vi "Acquisition Message Loop.vi"(8 "error in (no error)":errorcluster, 9 "queue out":refnum<queue>, 10 "Data Notifier":refnum<notifier>, 11 "Message Queues":T1) -> (0 "error out":errorcluster)   [LabVIEW 2022 SP3, in "Acquisition.lvlib"]
doc: "Message loop for handling messages pertaining to the acquisition of data from the hardware."
uses:
  Acquisition.lvlib
  support/Message Queue/Message Cluster.ctl
  Acquisition State.ctl
  GlobalVariable/GlobalDisconnected.vi
  GlobalVariable/GlobalFirstRep.vi
  GlobalVariable/GlobalPowerByTime.vi
  GlobalVariable/GlobalPosXbyTime.vi
  GlobalVariable/GlobalPosYbyTime.vi
  GlobalVariable/GlobalProfileByTime.vi
  GlobalVariable/GlobalTensionByTime.vi
  GlobalVariable/GlobalTemperatureByTime.vi
  GlobalVariable/Globalt0.vi
  support/Message Queue/Enqueue Message (Single).vi
  GlobalVariable/GlobalLongueurOnde.vi
  GlobalVariable/GlobalTimeStep.vi
  <vilib>/Utility/error.llb/Error Cluster From Error Code.vi
  <vilib>/ErrorRing/Error Ring.xnode
  support/Message Queue/Message Queue.lvlib
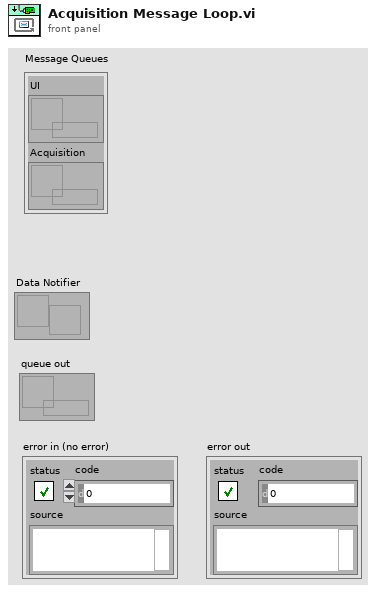
[diagram p1: front panel]
types:
  T1 = cluster{"UI":refnum<queue>, "Acquisition":refnum<queue>}
  T2 = enum16{"open", "replace", "create", "open or create", "replace or create", "replace or create with confirmation"}
  T3 = typedef "Acquisition.lvlib/Acquisition State.ctl" = enum16{"Idle", "Acquiring"}
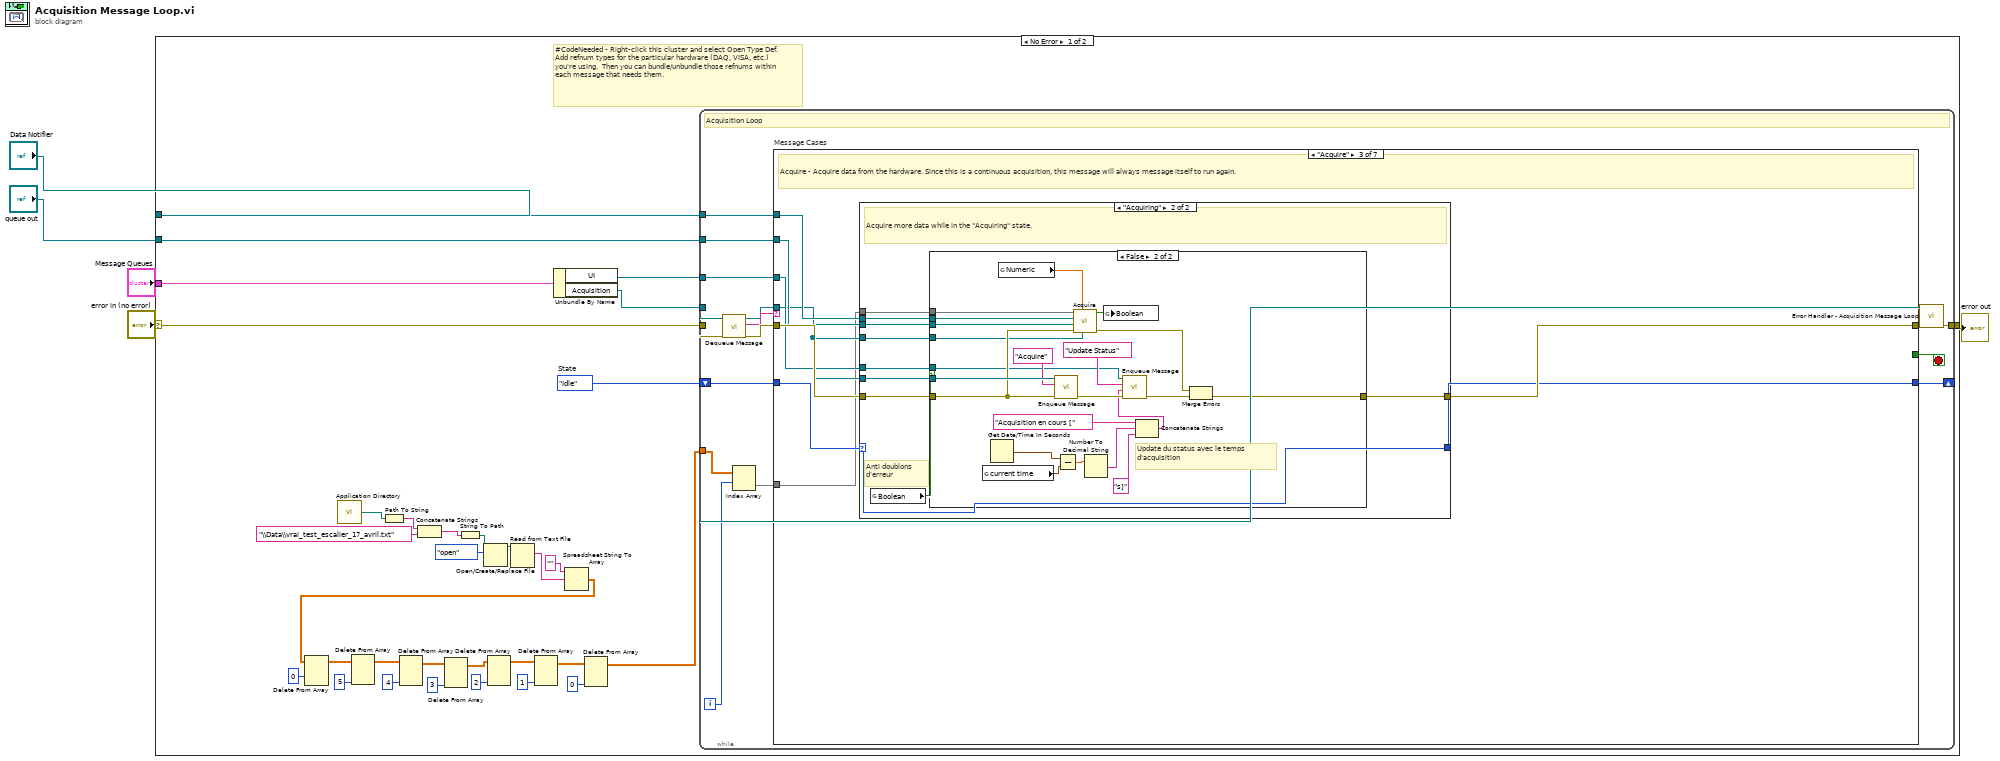
[diagram p0: block diagram]
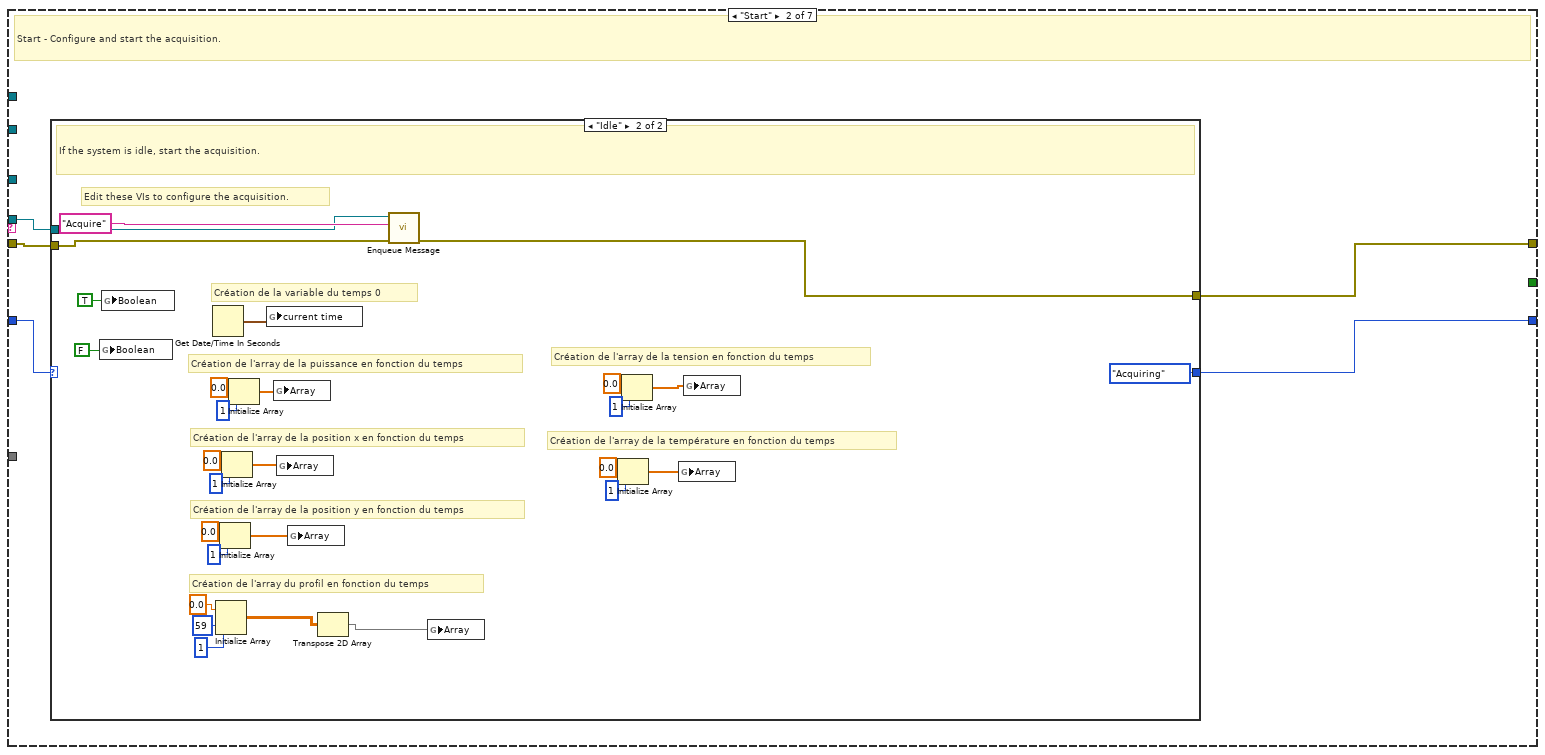
[diagram p3: hidden frame]
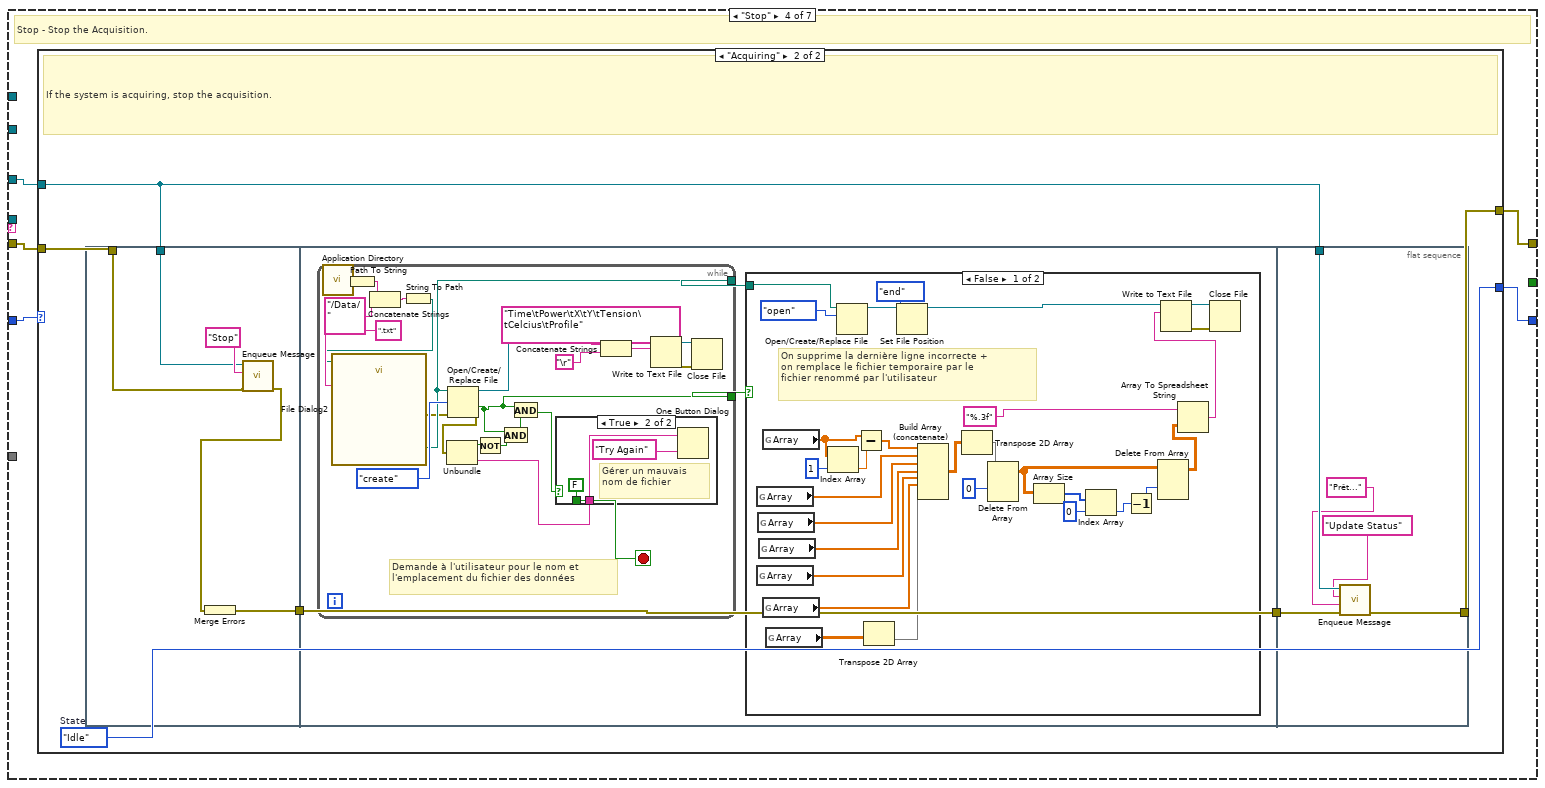
[diagram p7: hidden frame]
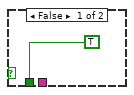
[diagram p10: hidden frame]
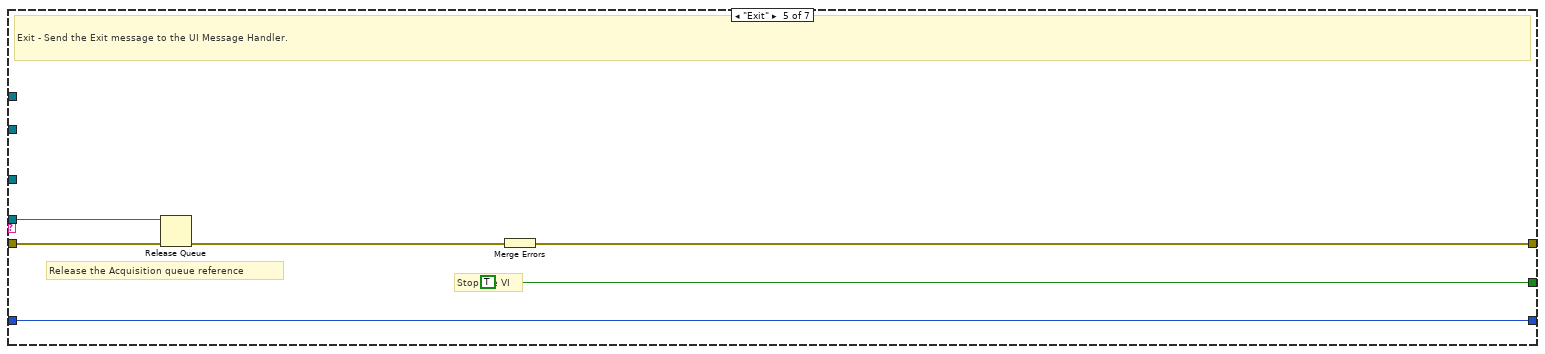
[diagram p11: hidden frame]
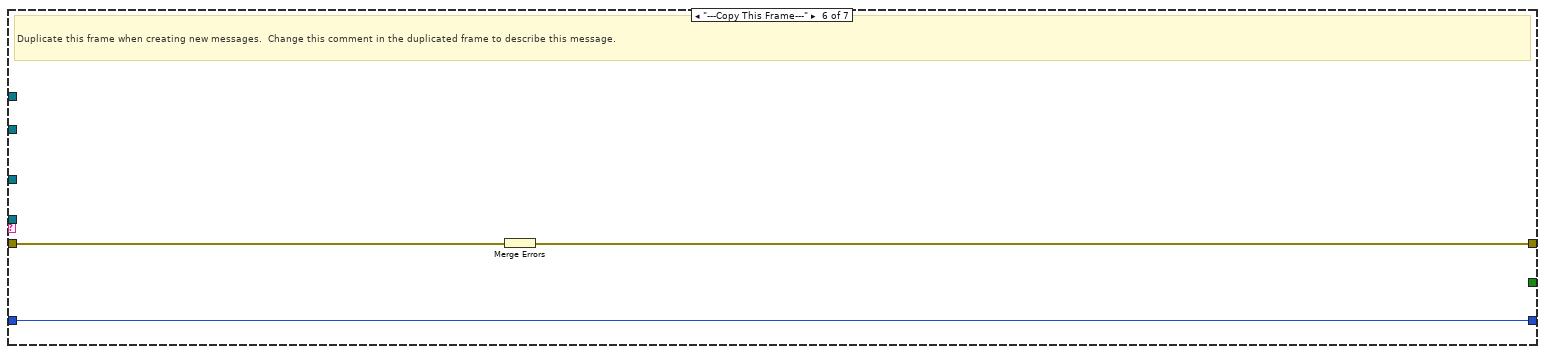
[diagram p12: hidden frame]
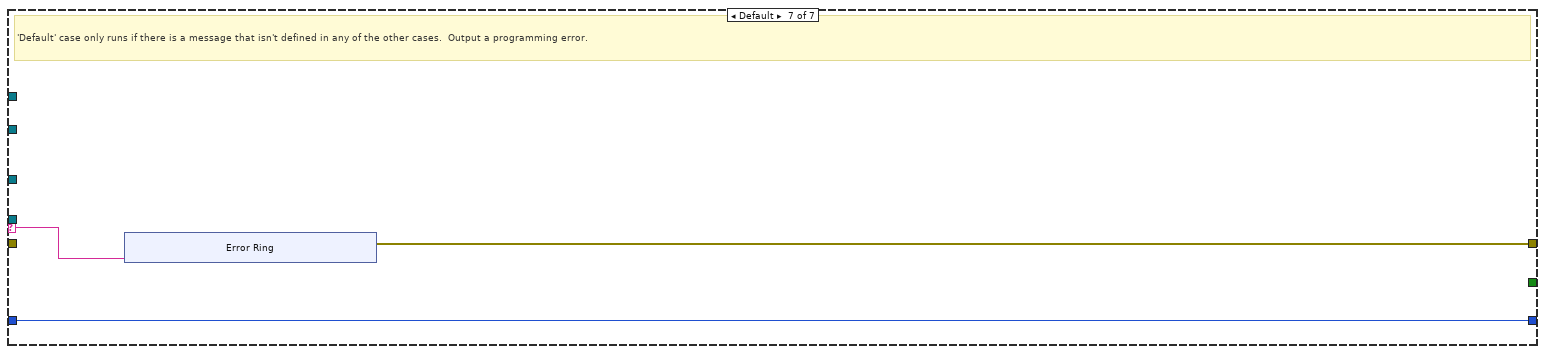
[diagram p13: hidden frame]
diagram:
  n1 = case shown="No Error" "error in (no error)" {
    selector: "error in (no error)" -> [w34 w236]
    tunnel: "Message Queues" -> [w37 _]
    tunnel: [w35 w236] -> w4
    tunnel: "Data Notifier" -> [w32 _]
    tunnel: "queue out" -> [w31 _]
    frame No Error {
      w30 = Acquisition_State."Idle"  # State
      # "#CodeNeeded - Right-click this cluster and select Open Type Def.  Add refnum types for the particular hardware (DAQ, VISA, etc.) you're using.  Then you can bundle/unbundle those refnums within each message that needs them."
      n2 = call <vilib>:"Application Directory.vi"() -> ("Application Directory"=w29:path)
      n3 = Path To String(path=w29) -> (string=w28:string)
      n4 = Concatenate Strings(w28, "\\Data\\vrai_test_escalier_17_avril.txt" ("string")) -> (w26:string)
      n5 = String To Path(string=w26) -> (path=w25:path)
      n6 = Open/Create/Replace File(file path (use dialog)=w25, operation (0:open)=T2."open") -> (refnum out=w23:refnum<file>)  [unwired: 4 in, 2 out]
      n7 = Read from Text File(file (use dialog)=w23) -> (text=w22:string)  [unwired: 3 in, 3 out]
      n8 = Unbundle By Name(w37) -> ("UI"=w33:refnum<queue>, "Acquisition"=w36:refnum<queue>)
      n9 = Spreadsheet String To Array(format string="", spreadsheet string=w22) -> (array=w7:dbl[][])  [unwired: 2 in]
      n10 = Delete From Array(array=w7, index (row)=0) -> (array with subset deleted=w19:dbl[][])  [unwired: 2 in, 1 out]
      n11 = Delete From Array(array=w19, index (col)=5 ("disabled index (col)")) -> (array with subset deleted=w17:dbl[][])  [unwired: 2 in, 1 out]
      n12 = Delete From Array(array=w17, index (col)=4 ("disabled index (col)")) -> (array with subset deleted=w15:dbl[][])  [unwired: 2 in, 1 out]
      n13 = Delete From Array(array=w15, index (col)=3 ("disabled index (col)")) -> (array with subset deleted=w12:dbl[][])  [unwired: 2 in, 1 out]
      n14 = Delete From Array(array=w12, index (col)=2) -> (array with subset deleted=w11:dbl[][])  [unwired: 2 in, 1 out]
      n15 = Delete From Array(array=w11, index (col)=1 ("disabled index (col)")) -> (array with subset deleted=w8:dbl[][])  [unwired: 2 in, 1 out]
      n16 = Delete From Array(array=w8, index (col)=0) -> (array with subset deleted=w6:dbl[][])  [unwired: 2 in, 1 out]
      n17 = while {
        tunnel: w36 -> [w41]
        tunnel: w33 -> [w42]
        tunnel: w32 -> [w49]
        tunnel: w31 -> [w48]
        shift-right: [w46] -> _
        shift-left: w30 -> [w47]
        tunnel: w34 -> [w52]
        tunnel: [w45] -> w35
        tunnel: w6 -> [w39]
        i -> [w40]
        stop <- w53 stop-if-true
        # "Acquisition Loop"
        n18 = call "Dequeue Message.vi"("error in (no error)"=w52, "Message Queue"=w41) -> ("error out"=w51:errorcluster, "Message"=w50:string, "dup Message Queue"=w43:refnum<queue>)  [unwired: 6 in, 1 out]
        n19 = Index Array(array=w39, index (row)=w40) -> (element=w38:dbl[])  [unwired: 1 in]
        n20 = case "Message Cases" shown="\"Acquire\"" w50 {
          selector: w50 -> [_ _ _ _ _ _ w226]
          tunnel: w43 -> [_ w58 w92 _ w218 _ _]
          tunnel: w51 -> [w55 w59 w98 w138 w220 w225 _]
          tunnel: [w55 w60 w99 w136 w221 w224 w227] -> w44
          tunnel: [_ _ _ _ TRUE _ _] -> w53
          tunnel: w42 -> [_ _ w93 w137 _ _ _]
          tunnel: w49 -> [_ _ w97 _ _ _ _]
          tunnel: w48 -> [_ _ w96 _ _ _ _]
          tunnel: w47 -> [w54 w56 w94 w139 w217 w223 w228]
          tunnel: [w54 w57 w95 w135 w217 w223 w228] -> w46
          tunnel: w38 -> [_ _ w91 _ _ _ _]
          frame "Initialize" {
            # "Initialize  - Initialize is currently a no-op.  The hardware initialization takes place in the 'Start' message."
          }
          frame "Start" {
            # "Start - Configure and start the acquisition."
            n21 = case shown="\"Idle\"" w56 {
              selector: w56 -> [w61 _]
              tunnel: [w62 w86] -> w60
              tunnel: w59 -> [w62 w90]
              tunnel: w58 -> [_ w87]
              tunnel: [w61 Acquisition_State."Acquiring" ("Acquisition State")] -> w57
              frame "Acquiring" {
                # "The system is already acquiring. Ignore the \"Start\" message."
              }
              frame "Idle" {
                # "Création de l'array de la température en fonction du temps"
                # "Création de l'array de la tension en fonction du temps"
                # "Création de la variable du temps 0"
                # "Création de l'array du profil en fonction du temps"
                # "Création de l'array de la position y en fonction du temps"
                # "Création de l'array de la position x en fonction du temps"
                # "Création de l'array de la puissance en fonction du temps"
                # "Edit these VIs to configure the acquisition."
                # "If the system is idle, start the acquisition."
                n22 = global write "GlobalDisconnected.vi" "Boolean"(FALSE) -> ()
                n23 = global write "GlobalFirstRep.vi" "Boolean"(TRUE ("Boolean")) -> ()
                n24 = Get Date/Time In Seconds() -> (seconds since 1Jan1904=w69:timestamp)
                n25 = Initialize Array(0.0, 59 ("dimension size"), 1 ("dimension size")) -> (w82:dbl[][])
                n26 = Initialize Array(0.0, 1) -> (w83:dbl[])
                n27 = Initialize Array(0.0, 1) -> (w84:dbl[])
                n28 = Initialize Array(0.0, 1) -> (w85:dbl[])
                n29 = global write "Globalt0.vi" "current time"(w69) -> ()
                n30 = global write "GlobalPowerByTime.vi" "Array"(w85) -> ()
                n31 = global write "GlobalPosXbyTime.vi" "Array"(w84) -> ()
                n32 = global write "GlobalPosYbyTime.vi" "Array"(w83) -> ()
                n33 = Transpose 2D Array(2D array=w82) -> (transposed array=w81:dbl[][])
                n34 = call-poly "Enqueue Message.vi"("error in (no error)"=w90, "Message"="Acquire", "Message Queue"=w87) -> ("error out"=w86:errorcluster)  [unwired: 7 in, 1 out]
                n35 = global write "GlobalProfileByTime.vi" "Array"(w81) -> ()
                n36 = Initialize Array(0.0, 1) -> (w63:dbl[])
                n37 = Initialize Array(0.0, 1) -> (w64:dbl[])
                n38 = global write "GlobalTemperatureByTime.vi" "Array"(w63) -> ()
                n39 = global write "GlobalTensionByTime.vi" "Array"(w64) -> ()
              }
            }
          }
          frame "Acquire" {
            # "Acquire - Acquire data from the hardware. Since this is a continuous acquisition, this message will always message itself to run again."
            n40 = case shown="\"Acquiring\"" w94 {
              selector: w94 -> [w100 w107]
              tunnel: [w101 w111] -> w99
              tunnel: w92 -> [_ w110]
              tunnel: w98 -> [w101 w106]
              tunnel: w97 -> [_ w109]
              tunnel: w96 -> [_ w108]
              tunnel: [w100 w107] -> w95
              tunnel: w93 -> [_ w105]
              tunnel: w92 -> [_ w104]
              tunnel: w91 -> [_ w102]
              frame "Idle" {
                # "Ignore \"Acquire\" messages when the acquisition is idle."
              }
              frame "Acquiring" {
                # "Anti doublons\nd'erreur"
                # "Acquire more data while in the \"Acquiring\" state."
                n41 = global read "GlobalDisconnected.vi" "Boolean"() -> (w103:bool)
                n42 = case shown="False" w103 {
                  tunnel: [w112 w134] -> w111
                  tunnel: w110 -> [_ w133]
                  tunnel: w109 -> [_ w130]
                  tunnel: w108 -> [_ w129]
                  tunnel: w106 -> [w112 w128]
                  tunnel: w105 -> [_ w117]
                  tunnel: w104 -> [_ w116]
                  tunnel: w102 -> [_ w113]
                  frame True {
                  }
                  frame False {
                    # "Update du status avec le temps\nd'acquisition"
                    n43 = global read "Globalt0.vi" "current time"() -> (w123:timestamp)
                    n44 = Get Date/Time In Seconds() -> (seconds since 1Jan1904=w122:timestamp)
                    n45 = global read "GlobalLongueurOnde.vi" "Numeric"() -> (w115:dbl)
                    n46 = call-poly "Enqueue Message.vi"("error in (no error)"=w128, "Message"="Acquire", "Message Queue"=w133) -> ("error out"=w126:errorcluster)  [unwired: 7 in, 1 out]
                    n47 = Subtract(x=w122, y=w123) -> (x-y=w124:dbl)
                    n48 = call "Acquire.vi"("Acquisition"=w116, "Longueur d'onde"=w115, "error in (no error)"=w128, "Data Queue"=w129, "Data Notifier"=w130, "Array"=w113) -> ("error out"=w132:errorcluster, "Disconnected"=w114:bool)  [unwired: 4 in]
                    n49 = Number To Decimal String(number=w124) -> (decimal integer string=w121:string)  [unwired: 1 in]
                    n50 = global write "GlobalDisconnected.vi" "Boolean"(w114) -> ()
                    n51 = Concatenate Strings("Acquisition en cours [", w121, "s]" ("string")) -> (w119:string)
                    n52 = call-poly "Enqueue Message.vi"("error in (no error)"=w126, "Message Data"=w119, "Message"="Update Status", "Message Queue"=w117) -> ("error out"=w127:errorcluster)  [unwired: 6 in, 1 out]
                    n53 = Merge Errors(w132, w127) -> (w134:errorcluster)
                  }
                }
              }
            }
          }
          frame "Stop" {
            # "Stop - Stop the Acquisition."
            n54 = case shown="\"Acquiring\"" w139 {
              selector: w139 -> [w141 _]
              tunnel: w138 -> [w140 w146]
              tunnel: w137 -> [_ w142]
              tunnel: [w140 w145] -> w136
              tunnel: [w141 w144] -> w135
              frame "Idle" {
                # "The system is already idle. Ignore the \"Stop\" message."
              }
              frame "Acquiring" {
                w144 = Acquisition_State."Idle"  # State
                # "If the system is acquiring, stop the acquisition."
                n55 = flat-sequence {
                  tunnel: [w152] -> w147
                  tunnel: w142 -> [w149]
                  tunnel: w146 -> [w148]
                  tunnel: w147 -> [w154]
                  tunnel: [w154] -> w143
                  tunnel: [w215] -> w145
                  tunnel: w143 -> [w216]
                  tunnel: w142 -> [w214]
                  frame #0 {
                    n56 = call-poly "Enqueue Message.vi"("error in (no error)"=w148, "Message"="Stop", "Message Queue"=w149) -> ("error out"=w151:errorcluster)  [unwired: 7 in, 1 out]
                    n57 = Merge Errors(w151) -> (w152:errorcluster)
                  }
                  frame #1 {
                    n58 = while {
                      tunnel: [w202] -> w155
                      tunnel: [w192] -> w153
                      stop <- w198 stop-if-true
                      # "Demande à l'utilisateur pour le nom et\nl'emplacement du fichier des données"
                      n59 = call <vilib>:"Application Directory.vi"() -> ("Application Directory"=w205:path)
                      n60 = Path To String(path=w205) -> (string=w206:string)
                      n61 = Concatenate Strings(w206, "/Data/") -> (w207:string)
                      n62 = String To Path(string=w207) -> (path=w191:path)
                      n63 = call "File Dialog2"("start path"=w191, "pattern (all files)"=".txt") -> ("selected path"=w202:path, "error out"=w200:errorcluster)  [unwired: 10 in, 2 out]
                      n64 = Open/Create/Replace File(file path (use dialog)=w202, error in=w200, operation (0:open)=T2."create") -> (refnum out=w187:refnum<file>, cancelled=w192:bool, error out=w197:errorcluster)  [unwired: 3 in]
                      n65 = Unbundle(w197) -> ("status"=w196:bool, "source"=w199:string)  [unwired: 1 out]
                      n66 = Not(x=w196) -> (.not. x?=w195:bool)
                      n67 = And(x=w192, y=w195) -> (x .and. y?=w194:bool)
                      n68 = And(x=w192, y=w194) -> (x .and. y?=w193:bool)
                      n69 = case shown="True" w193 {
                        tunnel: w199 -> [_ w211]
                        tunnel: [TRUE FALSE] -> w198
                        frame False {
                        }
                        frame True {
                          # "Gérer un mauvais \nnom de fichier"
                          n70 = One Button Dialog(message=w211, button name ("OK")="Try Again") -> ()  [unwired: 1 out]
                        }
                      }
                      n71 = Concatenate Strings("Time\tPower\tX\tY\tTension\tCelcius\tProfile", "\r") -> (w190:string)
                      n72 = Write to Text File(file (use dialog)=w187, text=w190) -> (refnum out=w186:refnum<file>, error out=w185:errorcluster)  [unwired: 2 in, 1 out]
                      n73 = Close File(refnum=w186, error in=w185) -> ()  [unwired: 2 out]
                    }
                    n74 = case shown="False" w153 {
                      tunnel: w155 -> [w178 _]
                      frame False {
                        # "On supprime la dernière ligne incorrecte + \non remplace le fichier temporaire par le \nfichier renommé par l'utilisateur"
                        n75 = global read "GlobalPowerByTime.vi" "Array"() -> (w177:dbl[])
                        n76 = global read "GlobalTensionByTime.vi" "Array"() -> (w157:dbl[])
                        n77 = global read "GlobalPosXbyTime.vi" "Array"() -> (w176:dbl[])
                        n78 = global read "GlobalPosYbyTime.vi" "Array"() -> (w175:dbl[])
                        n79 = global read "GlobalTimeStep.vi" "Array"() -> (w165:dbl[])
                        n80 = global read "GlobalTemperatureByTime.vi" "Array"() -> (w156:dbl[])
                        n81 = global read "GlobalProfileByTime.vi" "Array"() -> (w173:dbl[][])
                        n82 = Index Array(array=w165, index=1) -> (element=w166:dbl)
                        n83 = Open/Create/Replace File(file path (use dialog)=w178, operation (0:open)=T2."open") -> (refnum out=w182:refnum<file>)  [unwired: 4 in, 2 out]
                        n84 = Subtract(x=w165, y=w166) -> (x-y=w164:dbl[])
                        n85 = Transpose 2D Array(2D array=w173) -> (transposed array=w172:dbl[][])
                        n86 = Set File Position(refnum=w182, from (0:start)=enum16{"start", "end", "current"}."end") -> (refnum out=w184:refnum<file>)  [unwired: 2 in, 1 out]
                        n87 = Build Array (concatenate)(w164, w177, w176, w175, w157, w156, w172) -> (w174:dbl[][])
                        n88 = Transpose 2D Array(2D array=w174) -> (transposed array=w168:dbl[][])
                        n89 = Delete From Array(array=w168, index (row)=0) -> (array with subset deleted=w159:dbl[][])  [unwired: 2 in, 1 out]
                        n90 = Array Size(array=w159) -> (size(s)=w163:i32[])
                        n91 = Index Array(array=w163, index=0) -> (element=w161:i32)
                        n92 = Decrement(x=w161) -> (x-1=w160:i32)
                        n93 = Delete From Array(array=w159, index (row)=w160) -> (array with subset deleted=w158:dbl[][])  [unwired: 2 in, 1 out]
                        n94 = Array To Spreadsheet String(array=w158, 3:"%.3f" ("format string")) -> (spreadsheet string=w183:string)  [unwired: 1 in]
                        n95 = Write to Text File(file (use dialog)=w184, text=w183) -> (refnum out=w171:refnum<file>, error out=w170:errorcluster)  [unwired: 2 in, 1 out]
                        n96 = Close File(refnum=w171, error in=w170) -> ()  [unwired: 2 out]
                      }
                      frame True {
                      }
                    }
                  }
                  frame #2 {
                    n97 = call-poly "Enqueue Message.vi"("error in (no error)"=w216, "Message Data"="Prêt...", "Message"="Update Status", "Message Queue"=w214) -> ("error out"=w215:errorcluster)  [unwired: 6 in, 1 out]
                  }
                }
              }
            }
          }
          frame "Exit" {
            # "Release the Acquisition queue reference"
            # "Stop the VI"
            # "Exit - Send the Exit message to the UI Message Handler."
            n98 = Release Queue(queue=w218, error in (no error)=w220) -> (error out=w219:errorcluster)  [unwired: 1 in, 2 out]
            n99 = Merge Errors(w219) -> (w221:errorcluster)
          }
          frame "---Copy This Frame---" {
            # "Duplicate this frame when creating new messages.  Change this comment in the duplicated frame to describe this message."
            n100 = Merge Errors(w225) -> (w224:errorcluster)
          }
          frame Default {
            # "'Default' case only runs if there is a message that isn't defined in any of the other cases.  Output a programming error."
            n101 = xnode "Error Ring"("parameter 0"=w226) -> ("error out"=w227:errorcluster)
          }
        }
        n102 = call "Error Handler - Acquisition Message Loop.vi"("error in (no error)"=w44, "Message Queue"=w42) -> ("dup error in"=w45:errorcluster)  [unwired: 8 in, 1 out]
      }
    }
    frame Error {
    }
  }
  "error out" <- w4
